vi "取水点无水样数据存储.vi"(8 "error in (no error)":errorcluster, 9 "数据标识":string, 10 "数据类型":string, 11 "table":string) -> (0 "error out":errorcluster)   [LabVIEW 2016, in "PLC.lvlib"]
uses:
  PLC.lvlib
  <vilib>/Utility/sysdir.llb/System Directory Type.ctl
  <vilib>/addons/database/Connection.llb/DB Tools Open Connec (String).vi
  <vilib>/addons/database/NI_Database_API.lvlib
panel:
  in  "存储变量":T1={"时间标识"=timestamp(0 s since 1904-01-01), "测量模式"="", "数据类型"="N", "水样浓度值"=0.0, "数据标识"="Z", "LastTime"=timestamp(0 s since 1904-01-01)}
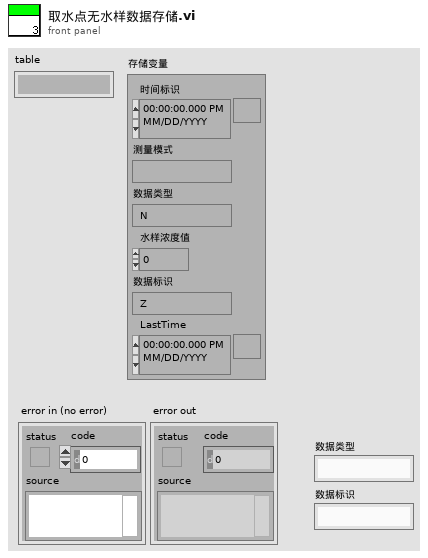
[diagram p1: front panel]
types:
  T1 = cluster{"时间标识":timestamp, "测量模式":string, "数据类型":string, "水样浓度值":dbl, "数据标识":string, "LastTime":timestamp}
  T2 = typedef "System Directory Type.ctl" = i32
  T3 = typedef "NI_Database_API.lvlib/Conn ObjectReference.ctl" = refnum<k1>
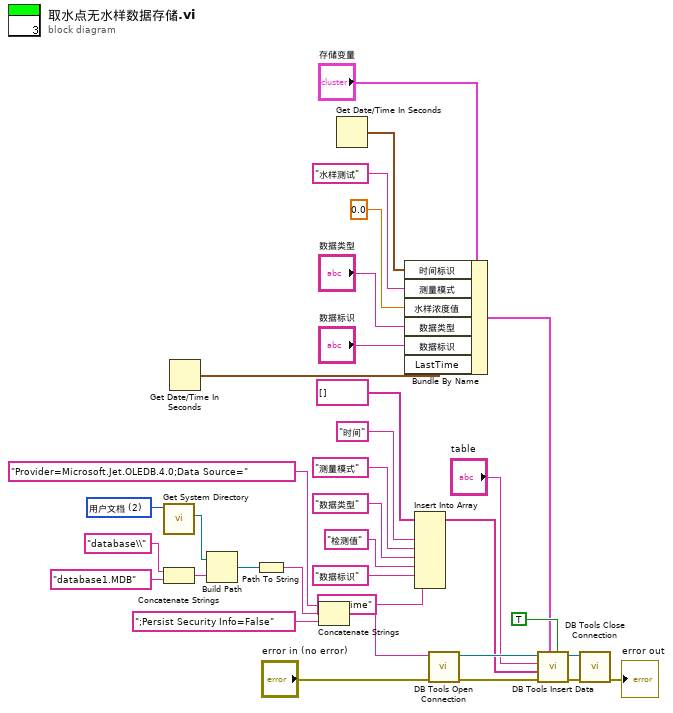
[diagram p0: block diagram]
diagram:
  w31 = T2 2 items=["用户目录"=0, "用户桌面"=1, "用户文档"=2, "用户应用程序数据"=3, "用户设置"=4, "用户临时目录"=5, "公共文档"=6, "公共应用程序数据"=7, "公共设置"=8, "公共缓存"=13, "系统核心库"=9, "系统安装库"=10, "应用程序文件"=11, "启动盘根目录"=12] ("system directory type")
  n1 = call <vilib>:"Get System Directory.vi"("system directory type"=w31) -> ("system directory"=w29:path)  [unwired: 10 in]
  n2 = Concatenate Strings("database\\" ("condition"), "database1.MDB" ("condition")) -> (w23:string)
  n3 = Get Date/Time In Seconds() -> (seconds since 1Jan1904=w1:timestamp)
  n4 = Build Path(base path=w29, name or relative path=w23) -> (appended path=w28:path)
  n5 = Path To String(path=w28) -> (string=w27:string)
  n6 = Concatenate Strings("Provider=Microsoft.Jet.OLEDB.4.0;Data Source=" ("condition"), w27, ";Persist Security Info=False" ("condition")) -> (w25:string)
  n7 = Get Date/Time In Seconds() -> (seconds since 1Jan1904=w6:timestamp)
  n8 = Bundle By Name(cluster="存储变量", "时间标识"=w6, "测量模式"="水样测试", "水样浓度值"=0.0, "数据类型"="数据类型", "数据标识"="数据标识", "LastTime"=w1) -> (w8:T1)
  n9 = Insert Into Array(array=string[] [] ("columns"), new element #1="时间" ("新元素/子数组"), new element #2="测量模式" ("新元素/子数组"), new element #3="数据类型" ("新元素/子数组"), new element #4="检测值" ("新元素/子数组"), new element #5="数据标识" ("新元素/子数组"), new element #6="LastTime" ("新元素/子数组")) -> (w15:string[])  [unwired: 1 in]
  n10 = call-poly <vilib>:"DB Tools Open Connection.vi"("error in (no error)"="error in (no error)", "connection information"=w25) -> ("error out"=w21:errorcluster, "connection reference"=w22:T3)  [unwired: 6 in]
  n11 = call <vilib>:"DB Tools Insert Data.vi"("create table? (F)"=TRUE, "data"=w8, "error in (no error)"=w21, "columns"=w15, "table"="table", "connection reference"=w22) -> ("error out"=w33:errorcluster, "connection reference out"=w34:T3)  [unwired: 4 in]
  n12 = call <vilib>:"DB Tools Close Connection.vi"("error in (no error)"=w33, "connection reference"=w34) -> ("error out"=→"error out":errorcluster)  [unwired: 5 in]
